vi "Curtin1_AdvancedPrefs.vi"(8 "Type":bool, 9 "Selection":T2(radio), 11 "Instrument:Test Name":string) -> (1 "Selection out":T1(ring), 3 "message":string)   [LabVIEW 2022 SP3]
panel:
  out "Generated Zip File":path
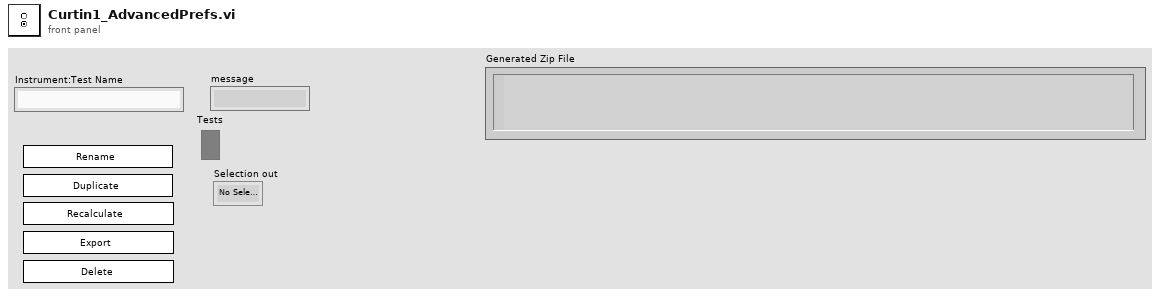
[diagram p1: front panel]
types:
  T1 = enum32{"No Selection", "Rename", "Recalculate", "Export", "Delete"}
  T2 = enum32{"No Selection", "Rename", "Recalculate", "Export", "Delete", "Duplicate"}
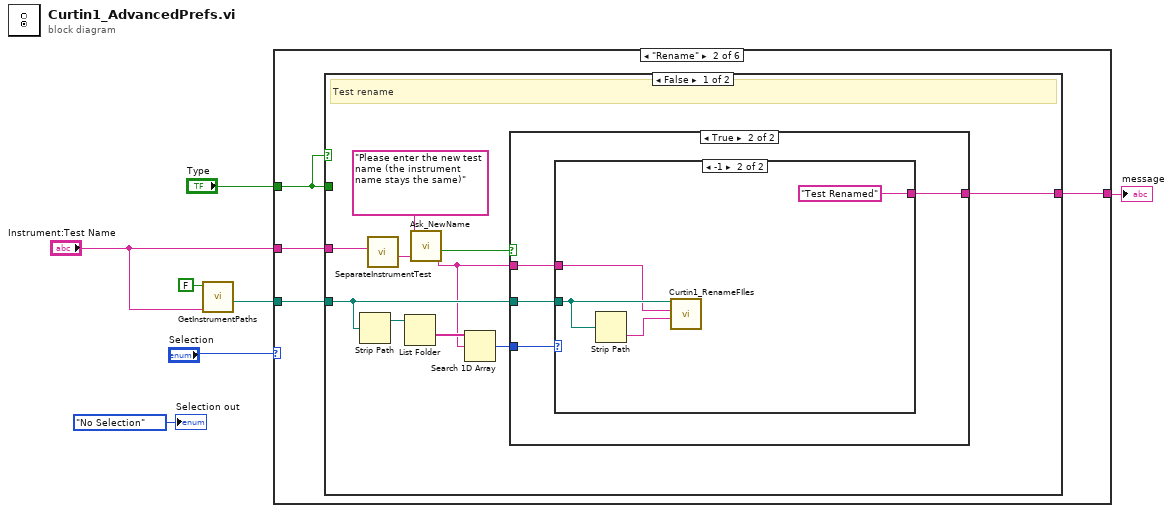
[diagram p0: block diagram]
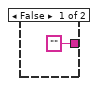
[diagram p3: hidden frame]
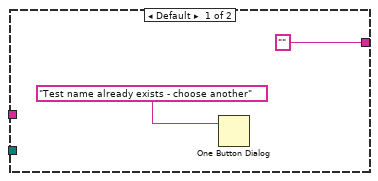
[diagram p4: hidden frame]
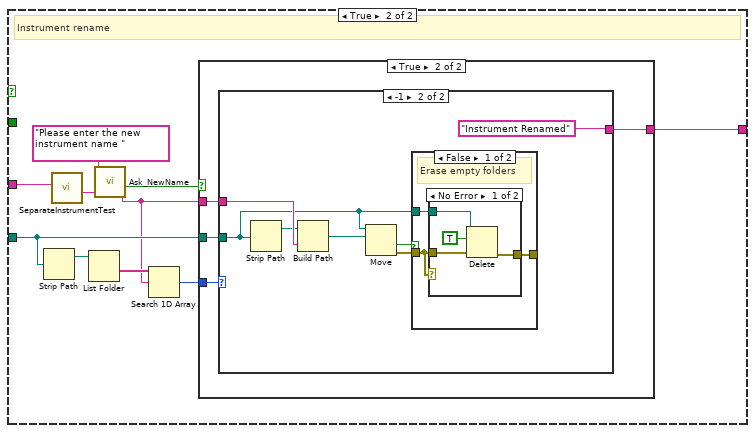
[diagram p5: hidden frame]
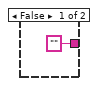
[diagram p6: hidden frame]
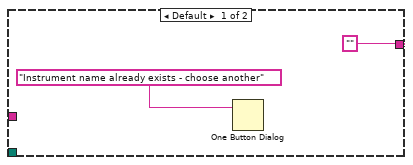
[diagram p7: hidden frame]
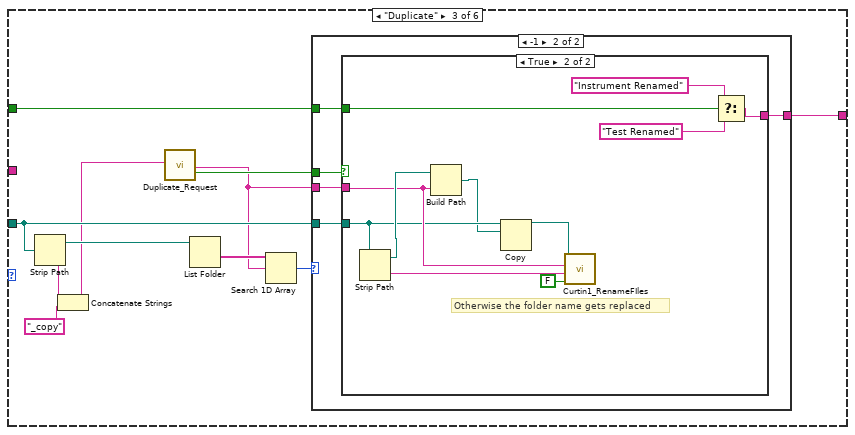
[diagram p10: hidden frame]
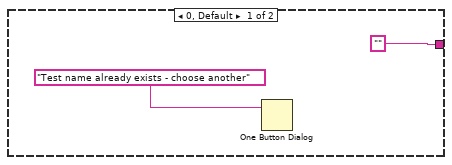
[diagram p11: hidden frame]
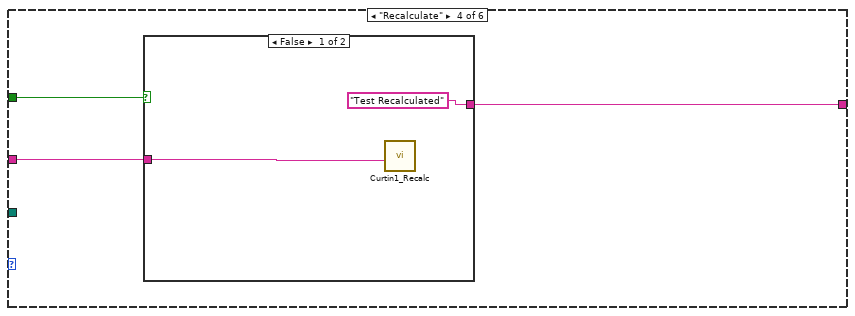
[diagram p13: hidden frame]
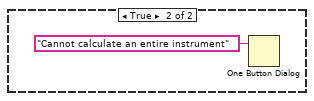
[diagram p14: hidden frame]
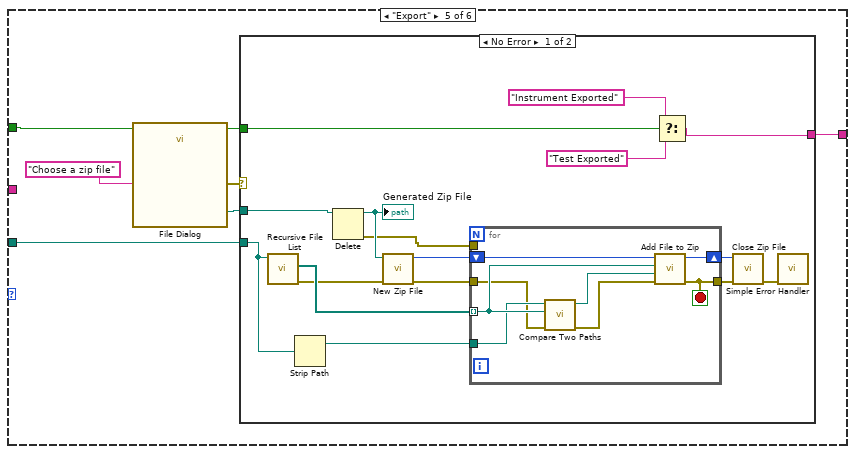
[diagram p15: hidden frame]
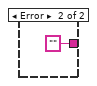
[diagram p16: hidden frame]
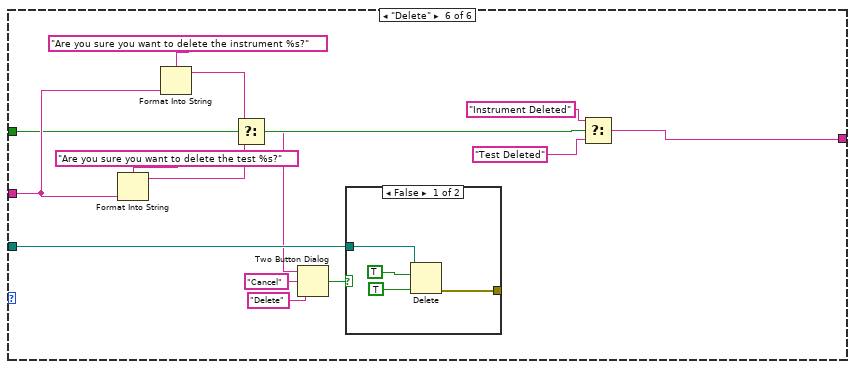
[diagram p17: hidden frame]
diagram:
  n1 = call "GetInstrumentPaths.vi"("Instrument"="Instrument:Test Name", "Build?"=FALSE) -> ("Path To Test Folder"=w5:path)  [unwired: 5 in, 4 out]
  n2 = case shown="\"Rename\"" "Selection" {
    tunnel: w5 -> [_ w10 w73 _ w103 w144]
    tunnel: "Instrument:Test Name" -> [_ w9 _ w96 _ w138]
    tunnel: [_ w11 w74 w94 w101 w140] -> w4
    tunnel: "Type" -> [_ w8 w68 w95 w102 w134]
    frame "No Selection", Default {
    }
    frame "Rename" {
      n3 = case shown="False" w8 {
        tunnel: [w21 w42] -> w11
        tunnel: w10 -> [w20 w41]
        tunnel: w8 -> [_ _]
        tunnel: w9 -> [w15 w36]
        frame False {
          # "Test rename"
          n4 = Strip Path(path=w20) -> (stripped path=w19:path)  [unwired: 1 out]
          n5 = call "SeparateInstrumentTest.vi"("Instrument"=w15) -> ("Just test"=w14:string)  [unwired: 6 in, 4 out]
          n6 = List Folder(path=w19) -> (folder names=w18:string[])  [unwired: 3 in, 3 out]
          n7 = call "Ask_NewName.vi"("New Name"=w14, "Label"="Please enter the new test name (the instrument name stays the same)") -> ("OK"=w12:bool, "New Name out"=w16:string)  [unwired: 8 in]
          n8 = Search 1D Array(1D array=w18, element=w16) -> (index of element=w17:i32)  [unwired: 1 in]
          n9 = case shown="True" w12 {
            tunnel: ["" ("message") w26] -> w21
            tunnel: w20 -> [_ w25]
            tunnel: w17 -> [_ w24]
            tunnel: w16 -> [_ w23]
            frame False {
            }
            frame True {
              n10 = case shown="-1" w24 {
                tunnel: ["" ("message") "Test Renamed" ("message")] -> w26
                tunnel: w25 -> [_ w31]
                tunnel: w23 -> [_ w30]
                frame Default {
                  n11 = One Button Dialog(message="Test name already exists - choose another") -> ()  [unwired: 1 in, 1 out]
                }
                frame -1 {
                  n12 = Strip Path(path=w31) -> (name=w29:string)  [unwired: 1 out]
                  n13 = call "Curtin1_RenameFIles.vi"("Old Name"=w29, "New Name"=w30, "Path To Test Folder"=w31) -> ()  [unwired: 9 in]
                }
              }
            }
          }
        }
        frame True {
          # "Instrument rename"
          n14 = Strip Path(path=w41) -> (stripped path=w40:path)  [unwired: 1 out]
          n15 = call "SeparateInstrumentTest.vi"("Instrument"=w36) -> ("Just test"=w35:string)  [unwired: 6 in, 4 out]
          n16 = List Folder(path=w40) -> (folder names=w39:string[])  [unwired: 3 in, 3 out]
          n17 = call "Ask_NewName.vi"("New Name"=w35, "Label"="Please enter the new instrument name ") -> ("OK"=w33:bool, "New Name out"=w37:string)  [unwired: 8 in]
          n18 = Search 1D Array(1D array=w39, element=w37) -> (index of element=w38:i32)  [unwired: 1 in]
          n19 = case shown="True" w33 {
            tunnel: ["" ("message") w47] -> w42
            tunnel: w41 -> [_ w46]
            tunnel: w38 -> [_ w45]
            tunnel: w37 -> [_ w44]
            frame False {
            }
            frame True {
              n20 = case shown="-1" w45 {
                tunnel: ["" ("message") "Instrument Renamed" ("message")] -> w47
                tunnel: w46 -> [_ w50]
                tunnel: w44 -> [_ w55]
                frame Default {
                  n21 = One Button Dialog(message="Instrument name already exists - choose another") -> ()  [unwired: 1 in, 1 out]
                }
                frame -1 {
                  n22 = Strip Path(path=w50) -> (stripped path=w54:path)  [unwired: 1 out]
                  n23 = Build Path(base path=w54, name or relative path=w55) -> (appended path=w53:path)
                  n24 = Move(source path=w50, 10:w53) -> (error out=w52:errorcluster, 1:w51:bool)  [unwired: 3 in, 1 out]
                  n25 = case shown="False" w51 {
                    tunnel: w52 -> [w58 _]
                    tunnel: [w59 _] -> _
                    tunnel: w50 -> [w57 _]
                    frame False {
                      # "Erase empty folders"
                      n26 = case shown="No Error" w58 {
                        tunnel: w58 -> [w63 w64]
                        tunnel: [w61 w64] -> w59
                        tunnel: w57 -> [w60 _]
                        frame No Error {
                          n27 = Delete(path (use dialog)=w60, entire hierarchy (F)=TRUE, error in=w63) -> (error out=w61:errorcluster)  [unwired: 2 in, 2 out]
                        }
                        frame Error {
                        }
                      }
                    }
                    frame True {
                    }
                  }
                }
              }
            }
          }
        }
      }
    }
    frame "Duplicate" {
      n28 = Strip Path(path=w73) -> (stripped path=w72:path, name=w67:string)
      n29 = Concatenate Strings(w67, "_copy" ("string")) -> (w65:string)
      n30 = call "Duplicate_Request.vi"("New Name"=w65) -> ("New Name"=w70:string, "OK"=w75:bool)  [unwired: 16 in, 1 out]
      n31 = List Folder(path=w72) -> (folder names=w71:string[])  [unwired: 3 in, 3 out]
      n32 = Search 1D Array(1D array=w71, element=w70) -> (index of element=w69:i32)  [unwired: 1 in]
      n33 = case shown="-1" w69 {
        tunnel: w75 -> [_ w82]
        tunnel: ["" ("message") w81] -> w74
        tunnel: w73 -> [_ w80]
        tunnel: w70 -> [_ w79]
        tunnel: w68 -> [_ w78]
        frame 0, Default {
          n34 = One Button Dialog(message="Test name already exists - choose another") -> ()  [unwired: 1 in, 1 out]
        }
        frame -1 {
          n35 = case shown="True" w82 {
            tunnel: w80 -> [_ w89]
            tunnel: w79 -> [_ w91]
            tunnel: [_ w84] -> w81
            tunnel: w78 -> [_ w87]
            frame False {
            }
            frame True {
              # "Otherwise the folder name gets replaced"
              n36 = Strip Path(path=w89) -> (stripped path=w93:path, name=w90:string)
              n37 = Build Path(base path=w93, name or relative path=w91) -> (appended path=w88:path)
              n38 = Copy(10:w88, 11:w89) -> (3:w92:path)  [unwired: 3 in, 2 out]
              n39 = call "Curtin1_RenameFIles.vi"("Files and folders?"=FALSE, "Old Name"=w90, "New Name"=w91, "Path To Test Folder"=w92) -> ()  [unwired: 8 in]
              n40 = Select(t="Instrument Renamed" ("message"), s=w87, f="Test Renamed" ("message")) -> (s? t:f=w84:string)
            }
          }
        }
      }
    }
    frame "Recalculate" {
      n41 = case shown="False" w95 {
        tunnel: w96 -> [w98 _]
        tunnel: ["Test Recalculated" ("message") _] -> w94
        frame False {
          n42 = call "Curtin1_Recalc.vi"("Instrument:Test Name"=w98) -> ()  [unwired: 11 in]
        }
        frame True {
          n43 = One Button Dialog(message="Cannot calculate an entire instrument") -> ()  [unwired: 1 in, 1 out]
        }
      }
    }
    frame "Export" {
      n44 = call "File Dialog"("prompt"="Choose a zip file") -> ("selected path"=w105:path, "error out"=w100:errorcluster)  [unwired: 11 in, 2 out]
      n45 = case shown="No Error" w100 {
        tunnel: w105 -> [w121 _]
        tunnel: w103 -> [w110 _]
        tunnel: w102 -> [w109 _]
        tunnel: [w106 "" ("message")] -> w101
        frame No Error {
          n46 = call <vilib>:"Recursive File List.vi"("Folder Path"=w110) -> ("error out"=w117:errorcluster, "All Files in Dir"=w118:path[])  [unwired: 6 in, 3 out]
          n47 = Strip Path(path=w110) -> (stripped path=w119:path)  [unwired: 1 out]
          n48 = Delete(path (use dialog)=w121) -> (deleted path=w120:path, error out=w111:errorcluster)  [unwired: 4 in, 1 out]
          "Generated Zip File" <- w120
          n49 = call <vilib>:"New Zip File.vi"("error in (no error)"=w117, "target"=w120) -> ("error out"=w114:errorcluster, "zip file out"=w113:i64)  [unwired: 1 in, 3 out]
          n50 = for {
            tunnel: w118 -> [w126] mode=indexing
            tunnel: w114 -> [w123]
            tunnel: [w127] -> w115
            shift-right: [w128] -> w116
            shift-left: w113 -> [w129]
            tunnel: w119 -> [w125]
            tunnel: w111 -> [_]
            stop <- w127 stop-if-true
            n51 = call <vilib>:"Compare Two Paths.vi"("error in (no error)"=w123, "Path 2"=w126, "Path 1"=w125) -> ("error out"=w122:errorcluster, "Relative Path from 1 to 2"=w124:path)  [unwired: 5 in, 2 out]
            n52 = call <vilib>:"Add File to Zip.vi"("error in (no error)"=w122, "destination path in zip"=w124, "source file path"=w126, "zip file in"=w129) -> ("error out"=w127:errorcluster, "zip file out"=w128:i64)  [unwired: 6 out]
          }
          n53 = Select(t="Instrument Exported" ("message"), s=w109, f="Test Exported" ("message")) -> (s? t:f=w106:string)
          n54 = call <vilib>:"Close Zip File.vi"("error in (no error)"=w115, "zip file in"=w116) -> ("error out"=w112:errorcluster)  [unwired: 1 in, 4 out]
          n55 = call <vilib>:"Simple Error Handler.vi"("error in (no error)"=w112) -> ()  [unwired: 1 in, 8 out]
        }
        frame Error {
        }
      }
    }
    frame "Delete" {
      n56 = Format Into String(format string="Are you sure you want to delete the test %s?" ("message"), w138) -> (resulting string=w135:string)  [unwired: 2 in, 1 out]
      n57 = Format Into String(format string="Are you sure you want to delete the instrument %s?" ("message"), w138) -> (resulting string=w136:string)  [unwired: 2 in, 1 out]
      n58 = Select(t=w136, s=w134, f=w135) -> (s? t:f=w133:string)
      n59 = Two Button Dialog(message=w133, 1:"Delete" ("F button name (\"Cancel\")"), 2:"Cancel" ("T button name (\"OK\")")) -> (T button?=w143:bool)
      n60 = case shown="False" w143 {
        tunnel: w144 -> [w146 _]
        tunnel: [w145 _] -> _
        frame False {
          n61 = Delete(path (use dialog)=w146, entire hierarchy (F)=TRUE, confirm (F)=TRUE) -> (error out=w145:errorcluster)  [unwired: 2 in, 2 out]
        }
        frame True {
        }
      }
      n62 = Select(t="Instrument Deleted" ("message"), s=w134, f="Test Deleted" ("message")) -> (s? t:f=w140:string)
    }
  }
  "message" <- w4
  "Selection out" <- T1."No Selection" ("Selection")
